vi "u8.array.to.u64.be.vi"(11 "data.u8.in":u8[](array[numeric])=[0, 0, 0, 0, 0, 0, 0, 0] format="%.0x") -> (3 "value.u64":u64 format="%.0x")   [LabVIEW 2020, in "fpganow.common.fpga.lvlib"]
uses:
  fpganow.common.fpga.lvlib
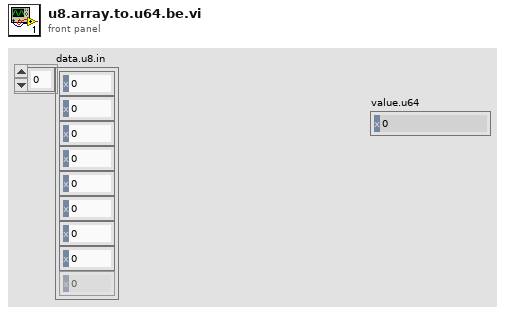
[diagram p1: front panel]
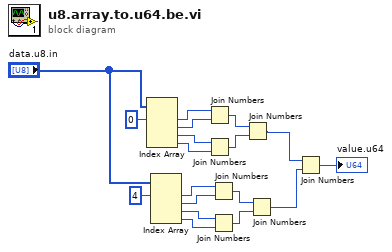
[diagram p0: block diagram]
diagram:
  n1 = Index Array(array="data.u8.in", index #1=0 ("index")) -> (element #1=w17:u8, element #2=w16:u8, element #3=w15:u8, element #4=w14:u8)  [unwired: 3 in]
  n2 = Index Array(array="data.u8.in", index #1=4 ("index")) -> (element #1=w9:u8, element #2=w8:u8, element #3=w7:u8, element #4=w6:u8)  [unwired: 3 in]
  n3 = Join Numbers(hi=w17, lo=w16) -> ((hi.lo)=w13:u16)
  n4 = Join Numbers(hi=w15, lo=w14) -> ((hi.lo)=w12:u16)
  n5 = Join Numbers(hi=w9, lo=w8) -> ((hi.lo)=w5:u16)
  n6 = Join Numbers(hi=w7, lo=w6) -> ((hi.lo)=w4:u16)
  n7 = Join Numbers(hi=w13, lo=w12) -> ((hi.lo)=w11:u32)
  n8 = Join Numbers(hi=w5, lo=w4) -> ((hi.lo)=w2:u32)
  n9 = Join Numbers(hi=w11, lo=w2) -> ((hi.lo)=→"value.u64":u64)
